vi "fgv_speed_cfg.vi"(7 "cmd":enum16{"write", "read"}(ring), 11 "speed cfg in":T1={"start heading adjust angular speed"=0.5, "move linear speed"=0.5, "decrease factor for linear speed"=80.0}) -> (3 "speed_cfg_out":T1)   [LabVIEW 2019]
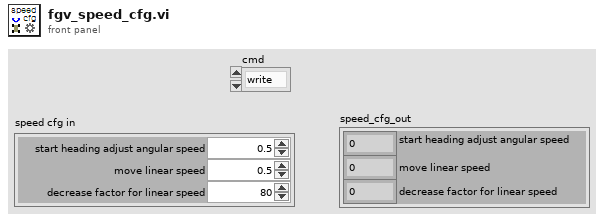
[diagram p1: front panel]
types:
  T1 = cluster{"start heading adjust angular speed":dbl, "move linear speed":dbl, "decrease factor for linear speed":dbl}
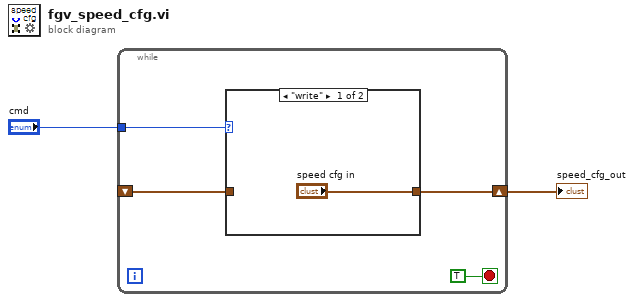
[diagram p0: block diagram]
diagram:
  n1 = while {
    tunnel: "cmd" -> [w5]
    shift-right: [w4] -> w1
    shift-left: _ -> [w3]
    stop <- TRUE stop-if-true
    n2 = case shown="\"write\"" w5 {
      tunnel: ["speed cfg in" w8] -> w4
      tunnel: w3 -> [_ w8]
      frame "write" {
      }
      frame "read", Default {
      }
    }
  }
  "speed_cfg_out" <- w1
